vi "Create Cal File Array (DAQ Rack).vi"() -> (3 "Cal Log OUT":string[][](array[string]))   [LabVIEW 2013]
uses:
  Type Defs/Units Type Def (DAQ Rack).ctl
  Type Defs/Channel Type Def (RIO).ctl
panel:
  in  "Channel to Cal":T1
  in  "Cal Unit":T2
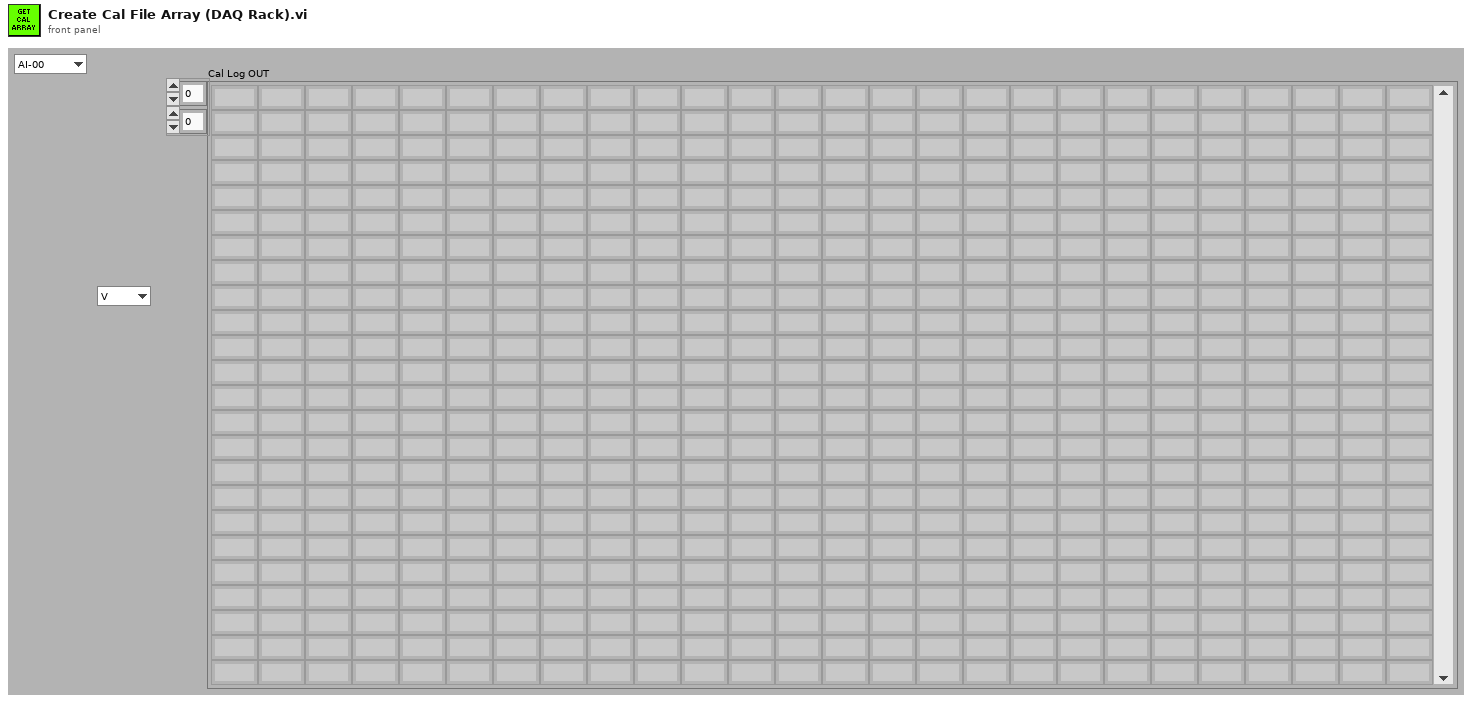
[diagram p1: front panel]
types:
  T1 = typedef "Channel Type Def (RIO).ctl" = enum16{"AI-00", "AI-01", "AI-02", "AI-03", "AI-04", "AI-05", "AI-06", "AI-07", "AI-08", "AI-09", "AI-10", "AI-11", "AI-12", "AI-13", "AI-14", "AI-15", "AI-16", "AI-17", "AI-18", "AI-19", "AI-20", "AI-21", "AI-22", "AI-23", "AI-24", "AI-25", "AI-26", "AI-27", "AI-28", "AI-29", "AI-30", "AI-31", "AI-32", "AI-33", "AI-34", "AI-35", "AI-36", "AI-37"}
  T2 = typedef "Units Type Def (DAQ Rack).ctl" = enum16{"V", "mA", "A", "Hz", "deg C"}
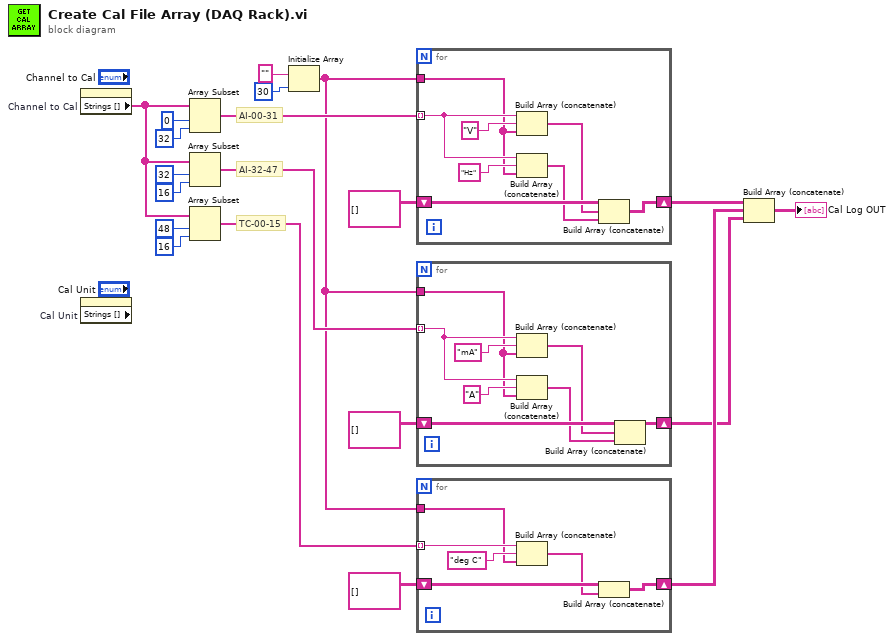
[diagram p0: block diagram]
diagram:
  # "TC-00-15"
  # "AI-32-47"
  # "AI-00-31"
  n1 = property on="Channel to Cal" class="Enum (strict)"() -> ("Strings []"=w1:string[])  [unwired: 2 in, 2 out]
  n2 = property on="Cal Unit" class="Enum (strict)" props=["Strings []"]() -> ()  [unwired: 2 in, 3 out]
  n3 = Array Subset(array=w1, index=0, length=32) -> (w14:string[])
  n4 = Array Subset(array=w1, index=32, length=16) -> (w9:string[])
  n5 = Array Subset(array=w1, index=48, length=16) -> (w3:string[])
  n6 = Initialize Array("", 30 ("dimension size")) -> (w2:string[])
  n7 = for {
    tunnel: w14 -> [w26] mode=indexing
    tunnel: w2 -> [w25]
    shift-right: [w23] -> w7
    shift-left: string[][] [] ("Cal Log OUT") -> [w24]
    n8 = Build Array (concatenate)(w26, "V", w25) -> (w22:string[])
    n9 = Build Array (concatenate)(w26, "Hz", w25) -> (w21:string[])
    n10 = Build Array (concatenate)(w24, w22, w21) -> (w23:string[][])
  }
  n11 = for {
    tunnel: w9 -> [w32] mode=indexing
    tunnel: w2 -> [w29]
    shift-right: [w35] -> w5
    shift-left: string[][] [] ("Cal Log OUT") -> [w36]
    n12 = Build Array (concatenate)(w32, "mA", w29) -> (w31:string[])
    n13 = Build Array (concatenate)(w32, "A", w29) -> (w30:string[])
    n14 = Build Array (concatenate)(w36, w31, w30) -> (w35:string[][])
  }
  n15 = for {
    tunnel: w3 -> [w41] mode=indexing
    tunnel: w2 -> [w40]
    shift-right: [w38] -> w6
    shift-left: string[][] [] ("Cal Log OUT") -> [w39]
    n16 = Build Array (concatenate)(w41, "deg C", w40) -> (w37:string[])
    n17 = Build Array (concatenate)(w39, w37) -> (w38:string[][])
  }
  n18 = Build Array (concatenate)(w7, w6, w5) -> (→"Cal Log OUT":string[][])
